vi "RRTAlgorithm2.vi"(0 "Dest x,y":dbl[](array[numeric]), 1 "Robot":T1={"id"=0, "function"=enum."Attacker", "x"=0.0, "y"=0.0, "orientation"=0.0, "v_tangent"=0.0, "v_normal"=0.0, "v_ang"=0.0, "kick_x"=0.0, "kick_z"=0.0, "dribble"=FALSE, "Timestamp"=timestamp(0 s since 1904-01-01), "estimatives"={"est_v_tangent"=0.0, "est_v_normal"=0.0, "est_vx"=0.0, "est_vy"=0.0, "Pos Robot Est"=[], "est_v_ang"=0.0}, "dest_x_kick"=0.0, "dest_y_kick"=0.0, "Gap Coord"=[], "States"=enum."Pass", "Path "=[], "Path  Smooth"=[], "Dest"=[], "vx_desired"=0.0, "vy_desired"=0.0, "slowBehavior"=FALSE, "VSSStates"=enum."Pass", "robotKickState"=enum."none", "role"=enum."DefenderArea"}, 2 "WayPointProb":dbl, 3 "Path in \n(Smooth do Feedback Node)":dbl[][](array[numeric]), 4 "Step":dbl, 5 "GoalProb":dbl, 6 "Simple Path":dbl[][](array[numeric]), 7 "Ball":T10, 8 "Initial Pos x,y":dbl[](array[numeric]), 9 "our_robots":T1[](array[typedef]), 10 "Initial Pos 1,x,y,0":dbl[](array[numeric]), 11 "enemy_robots":T1[](array[typedef]), 12 "ignoreBall?":bool, 13 "Field Geomtery":u32[](array[numeric]), 14 "AttackerAvoidArea":bool=TRUE, 19 "buffer":dbl[](array[numeric])) -> (16 "Path":dbl[][](array[numeric]))   [LabVIEW 2020]
uses:
  Vision_class/Old vision/SSL Detection Frame Simple Estimator Cameras VelCmd Folder/Core/AI Ball.ctl
  Vision_class/Old vision/Controls/AI Robot.ctl
  Vision_class/Old vision/Controls/Functions Enum.ctl
  Controls/estimatives.ctl
  Vision_class/Old vision/Controls/AttackerStates.ctl
  Vision_class/Old vision/Controls/PathDests.ctl
  Vision_class/Old vision/Controls/PathDest.ctl
  Navigation/VSSNavigation/VSSAttackerStates.ctl
  Robot_class/robotKickToStates.ctl
  Robot_class/roles.ctl
  <vilib>/Analysis/_algsub.llb/Real Vector Norm.vi
  <vilib>/Analysis/coordinate.llb/2D Cartesian Coordinate Rotation (Scalar).vi
  <vilib>/Analysis/NI_AALPro.lvlib
panel:
  out "useSimplePath":i32
  out "pathsize":i32
  out "debug":sgl
  out "newTree":dbl[](array[numeric])
  in  "threshold":dbl=80.0
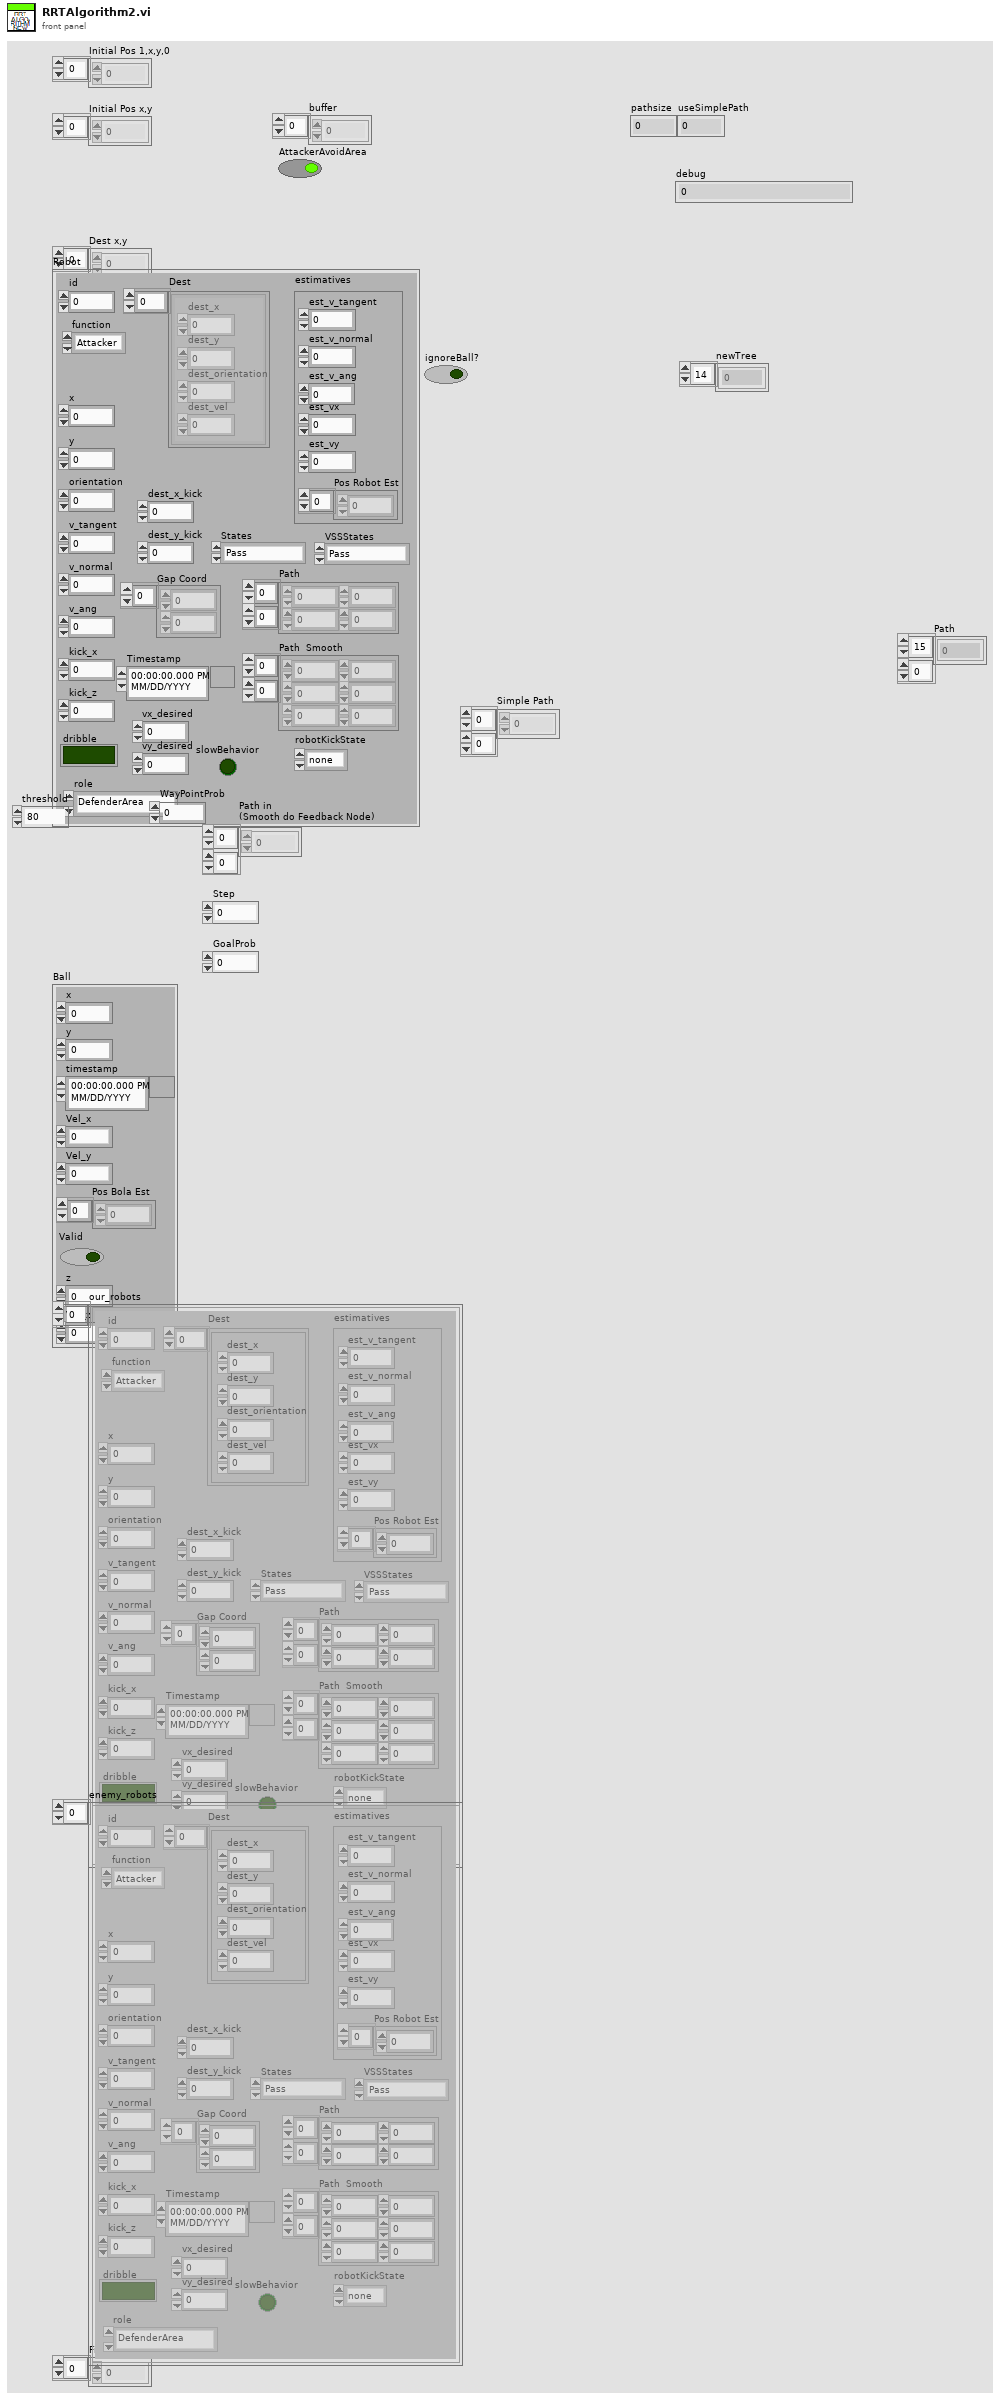
[diagram p1: front panel]
types:
  T1 = typedef "AI Robot.ctl" = cluster{"id":u32, "function":T2, "x":dbl, "y":dbl, "orientation":dbl, "v_tangent":dbl, "v_normal":dbl, "v_ang":dbl, "kick_x":dbl, "kick_z":dbl, "dribble":bool, "Timestamp":timestamp, "estimatives":T3, "dest_x_kick":dbl, "dest_y_kick":dbl, "Gap Coord":dbl[], "States":T4, "Path ":dbl[][], "Path  Smooth":dbl[][], "Dest":T5, "vx_desired":dbl, "vy_desired":dbl, "slowBehavior":bool, "VSSStates":T7, "robotKickState":T8, "role":T9}
  T2 = typedef "Functions Enum.ctl" = enum16{"2nd Striker", "Attacker", "Goalie", "Defender", "Striker", "Goto 0", "Dummy", "Kicker", "ZigZag 0", "ZigZag 1", "ZigZag 2", "ZigZag 3", "ZigZag 4", "ZigZag 5", "ZigZag 6", "ZigZag 7", "ZigZag 8", ""}
  T3 = typedef "estimatives.ctl" = cluster{"est_v_tangent":dbl, "est_v_normal":dbl, "est_vx":dbl, "est_vy":dbl, "Pos Robot Est":dbl[], "est_v_ang":dbl}
  T4 = typedef "AttackerStates.ctl" = enum16{"Pass", "GoToTangent", "BallGetting", "GoToKick", ""}
  T5 = typedef "PathDests.ctl" = T6[]
  T6 = typedef "PathDest.ctl" = cluster{"dest_x":dbl, "dest_y":dbl, "dest_orientation":dbl, "dest_vel":dbl}
  T7 = typedef "VSSAttackerStates.ctl" = enum16{"Pass", "GoToTangent", "BallGetting", "GoToKick", "Rotate anti-clockwise", "Rotate Clockwise", ""}
  T8 = typedef "robotKickToStates.ctl" = enum16{"shootFromDirect", "avoidCollideBall", "goToBackBall", "none", "walk", "turn", "oldKickToShoot", "oldKickToGoToBackBall", "shoot"}
  T9 = typedef "roles.ctl" = enum16{"SimpleBallPlacement", "BallPlacementAllyPasser", "BallPlacementAllyReceiver", "BallPlacementEnemy", "5Robots5th", "PassBestReceiver", "5Robots4th", "5Robots3rd", "5Robots2nd", "5Robots1st", "PassBestRobot", "WaitPass", "ABCThirdKicker", "ABCFirstKicker", "ABCSecondKicker", "Tabler", "TableFinalizer", "PrepareRollToPassRoller", "PrepareRollToPassReceiver", "SimplePassRoll", "SimplePassRollReceiver", "PenaltyDefense", "PreparePassReceiver 2", "PreparePassReceiver 1", "PassObserver", "Timeout", "Goto", "ZigZag", "None", "BallOutOfField", "DefenderArea", "Duelist", "AttackerStop", "FollowAttacker", "KeeperRole", "KickPenalty", "AttackerAimGoal", "AttackerBlock", "Marker", "Halt", "Shoot", "PassKicker", "PassReceiver", "TestRole", "PenaltyAttacker"}
  T10 = typedef "AI Ball.ctl" = cluster{"x":dbl, "y":dbl, "timestamp":timestamp, "Vel_x":dbl, "Vel_y":dbl, "Pos Bola Est":dbl[], "Valid":bool, "z":dbl, "Vel_z":dbl}
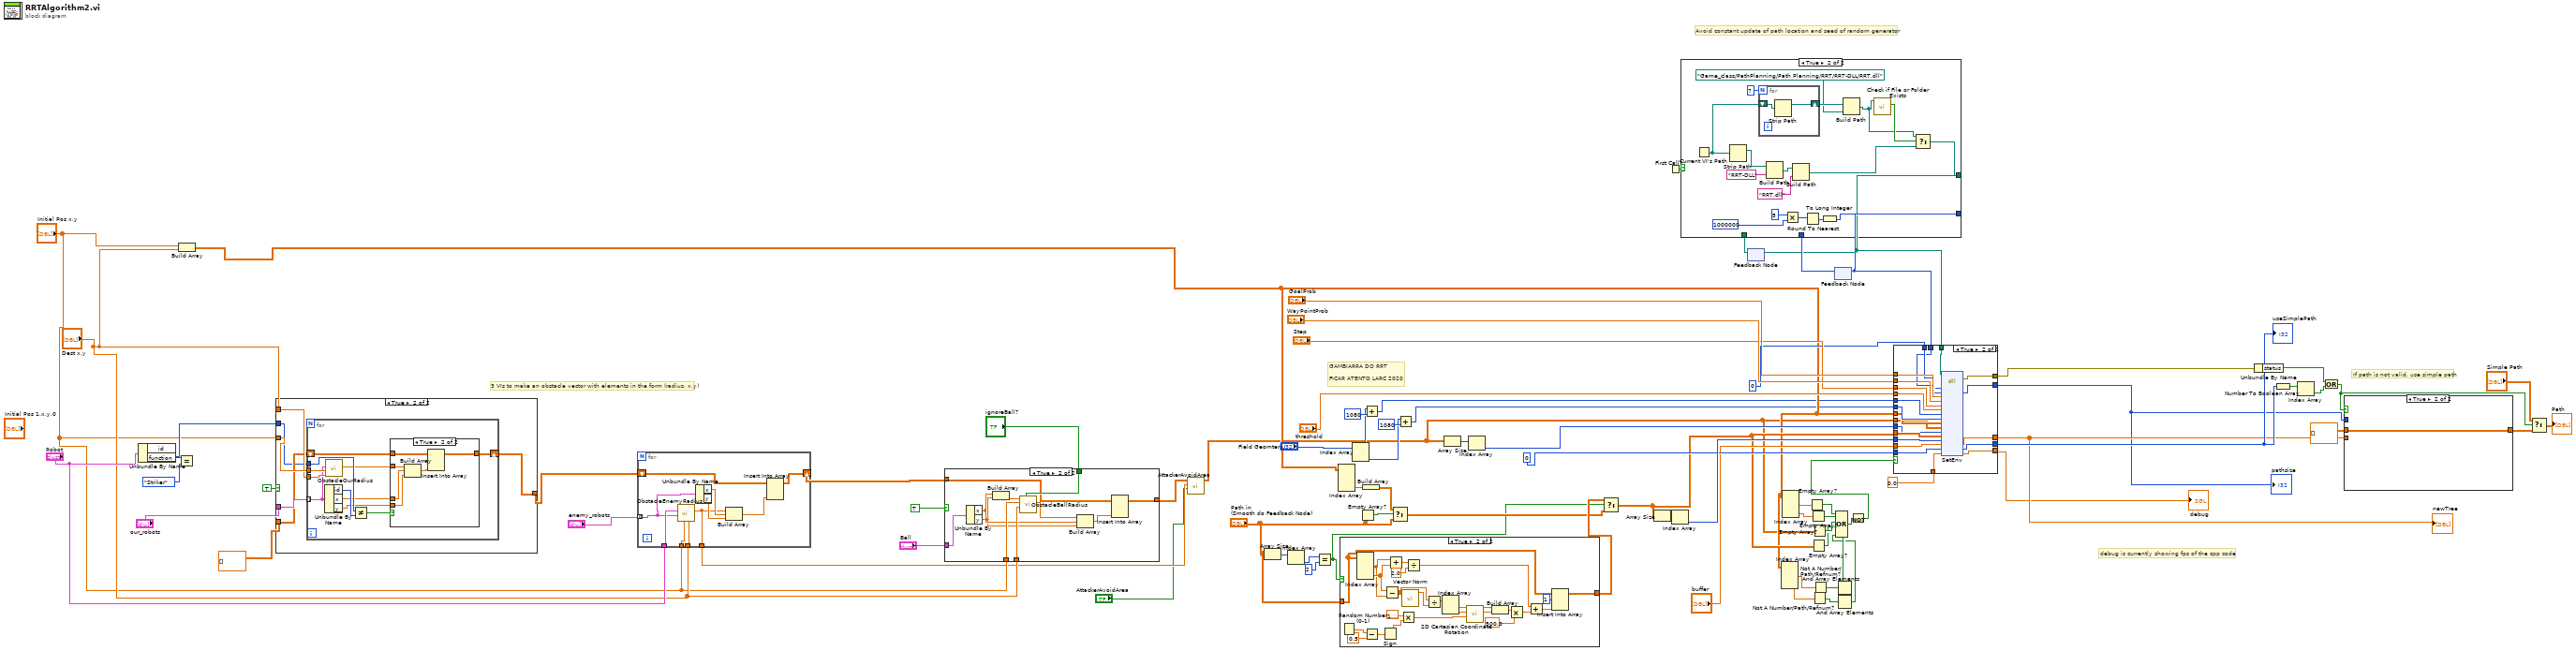
[diagram p0: block diagram]
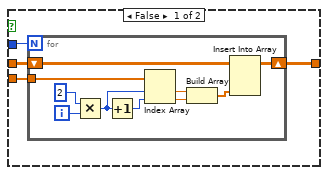
[diagram p4: hidden frame]
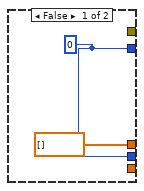
[diagram p5: hidden frame]
diagram:
  # "GAMBIARRA DO RRT\n\nFICAR ATENTO LARC 2020"
  # "debug is currently showing fps of the cpp code"
  # "If path is not valid, use simple path"
  # "3 VIs to make an obstacle vector with elements in the form (radius, x,y)"
  # "Avoid constant update of path location and seed of random generator"
  n1 = Unbundle By Name("Robot") -> ("id"=w69:u32, "function"=w73:T2)
  n2 = Equal?(x=w73, y=Functions_Enum."Striker" ("function")) -> ()  [unwired: 1 out]
  n3 = Build Array("Initial Pos x,y", "Dest x,y") -> (w12:dbl[][])
  n4 = case shown="True" TRUE {
    tunnel: "our_robots" -> [_ w89]
    tunnel: "Initial Pos x,y" -> [_ w88]
    tunnel: "Dest x,y" -> [_ w87]
    tunnel: dbl[][] [] ("appended array") -> [w83 w86]
    tunnel: [w83 w84] -> w66
    tunnel: w69 -> [_ w85]
    frame False {
    }
    frame True {
      n5 = for {
        tunnel: w89 -> [w98] mode=indexing
        tunnel: w88 -> [w100]
        tunnel: w87 -> [w99]
        shift-right: [w90] -> w84
        shift-left: w86 -> [w94]
        tunnel: w85 -> [w96]
        n6 = Unbundle By Name(w98) -> ("id"=w97:u32, "x"=w92:dbl, "y"=w91:dbl)
        n7 = call "ObstacleOurRadius.vi"("Goal"=w99, "Initial State"=w100, "other robot"=w98) -> ("obstacle enemy radius"=w93:dbl)  [unwired: 8 in]
        n8 = Not Equal?(x=w96, y=w97) -> (x != y?=w95:bool)
        n9 = case shown="True" w95 {
          tunnel: w94 -> [w101 w104]
          tunnel: [w101 w102] -> w90
          tunnel: w93 -> [_ w107]
          tunnel: w92 -> [_ w106]
          tunnel: w91 -> [_ w105]
          frame False {
          }
          frame True {
            n10 = Build Array(w107, w106, w105) -> (w103:dbl[])
            n11 = Insert Into Array(array=w104, new element=w103) -> (w102:dbl[][])  [unwired: 2 in]
          }
        }
      }
    }
  }
  n12 = for {
    tunnel: "enemy_robots" -> [w114] mode=indexing
    tunnel: "Initial Pos x,y" -> [w117]
    tunnel: "Dest x,y" -> [w116]
    tunnel: "Robot" -> [w115]
    shift-right: [w109] -> w62
    shift-left: w66 -> [w111]
    tunnel: [w108] -> w2
    n13 = call "ObstacleEnemyRadius.vi"("Goal"=w116, "Initial State"=w117, "Robot enemy"=w114, "Robot in"=w115) -> ("obstacle enemy radius"=w108:dbl)  [unwired: 7 in]
    n14 = Unbundle By Name(w114) -> ("x"=w113:dbl, "y"=w112:dbl)
    n15 = Build Array(w108, w113, w112) -> (w110:dbl[])
    n16 = Insert Into Array(array=w111, new element=w110) -> (w109:dbl[][])  [unwired: 2 in]
  }
  n17 = case shown="True" TRUE {
    tunnel: "Ball" -> [_ w129]
    tunnel: "Initial Pos x,y" -> [_ w127]
    tunnel: "Dest x,y" -> [_ w126]
    tunnel: "ignoreBall?" -> [_ w125]
    tunnel: w62 -> [w118 w124]
    tunnel: [w118 w123] -> w3
    frame False {
    }
    frame True {
      n18 = Unbundle By Name(w129) -> ("x"=w121:dbl, "y"=w120:dbl)
      n19 = Build Array(w121, w120) -> (w128:dbl[])
      n20 = call "ObstacleBallRadius.vi"("ignoreBall?"=w125, "Goal"=w126, "Initial State"=w127, "ball"=w128) -> ("obstacle enemy radius"=w122:dbl)  [unwired: 7 in]
      n21 = Build Array(w122, w121, w120) -> (w119:dbl[])
      n22 = Insert Into Array(array=w124, new element=w119) -> (w123:dbl[][])  [unwired: 2 in]
    }
  }
  n23 = call "AttackerAvoidArea.vi"("AttackerAvoidArea"="AttackerAvoidArea", "obstacle enemy radius"=w2, "array in"=w3) -> ("array out"=w4:dbl[][])  [unwired: 8 in]
  n24 = Array Size(array="Path in \n(Smooth do Feedback Node)") -> (size(s)=w40:i32[])
  n25 = Index Array(array=w40) -> (element=w39:i32)  [unwired: 1 in]
  n26 = Equal?(x=w39, y=2) -> (x = y?=w34:bool)
  n27 = Index Array(array=w12) -> (element #2=w57:dbl[])  [unwired: 4 in, 1 out]
  n28 = case shown="True" w34 {
    tunnel: "Path in \n(Smooth do Feedback Node)" -> [w130 w137]
    tunnel: [w130 w134] -> w36
    frame False {
    }
    frame True {
      n29 = Random Number (0-1)() -> (number: 0 to 1=w131:dbl)
      n30 = Index Array(array=w137) -> (element #1=w152:dbl[], element #2=w153:dbl[])  [unwired: 4 in]
      n31 = Subtract(x=w131, y=0.5) -> (x-y=w133:dbl)
      n32 = Sign(1:w133) -> (0:w148:dbl)
      n33 = Subtract(x=w153, y=w152) -> (x-y=w150:dbl[])
      n34 = Add(x=w152, y=w153) -> (x+y=w155:dbl[])
      n35 = Multiply(x=1.5707963267948966, y=w148) -> (x*y=w147:dbl)
      n36 = call-poly <vilib>:"Vector Norm.vi"("Input Vector"=w150) -> ("norm"=w151:dbl)  [unwired: 9 in, 1 out]
      n37 = Divide(x=w155, y=2.0) -> (x/y=w138:dbl[])
      n38 = Divide(x=w150, y=w151) -> (x/y=w146:dbl[])
      n39 = Index Array(array=w146) -> (element #1=w145:dbl, element #2=w144:dbl)  [unwired: 2 in]
      n40 = call-poly <vilib>:"2D Cartesian Coordinate Rotation.vi"("theta"=w147, "y"=w144, "x"=w145) -> ("y out"=w142:dbl, "x out"=w143:dbl)  [unwired: 6 in, 1 out]
      n41 = Build Array(w143, w142) -> (w140:dbl[])
      n42 = Multiply(x=w140, y=500.0) -> (x*y=w139:dbl[])
      n43 = Add(x=w138, y=w139) -> (x+y=w135:dbl[])
      n44 = Insert Into Array(array=w137, index (row)=1, new element=w135) -> (w134:dbl[][])  [unwired: 1 in]
    }
  }
  n45 = Index Array(array="Field Geomtery") -> (element #1=w7:u32, element #2=w10:u32)  [unwired: 2 in]
  n46 = Empty Array?(array="Path in \n(Smooth do Feedback Node)") -> (empty?=w58:bool)
  n47 = Build Array(w57) -> (w50:dbl[][])
  n48 = Add(x=w7, y=u32 1080) -> (x+y=w6:u32)
  n49 = Select(t=w50, s=w58, f="Path in \n(Smooth do Feedback Node)") -> (s? t:f=w35:dbl[][])
  n50 = Add(x=w10, y=u32 1080) -> (x+y=w9:u32)
  n51 = Array Size(array=w4) -> (size(s)=w60:i32[])
  n52 = Index Array(array=w60) -> (element=w76:i32)  [unwired: 1 in]
  n53 = Select(t=w36, s=w34, f=w35) -> (s? t:f=w30:dbl[][])
  n54 = Array Size(array=w30) -> (size(s)=w59:i32[])
  n55 = First Call?() -> (First Call?: T/F=w47:bool)
  n56 = Index Array(array=w59) -> (element=w78:i32)  [unwired: 1 in]
  n57 = feedback #1() -> (w46:path)  [unwired: 1 in]
  n58 = Index Array(array=w12) -> (element #1=w19:dbl[], element #2=w18:dbl[])  [unwired: 4 in]
  n59 = Index Array(array=w12) -> (element #1=w32:dbl[], element #2=w31:dbl[])  [unwired: 4 in]
  n60 = Empty Array?(array=w32) -> (empty?=w21:bool)
  n61 = Empty Array?(array=w31) -> (empty?=w20:bool)
  n62 = Empty Array?(array=w30) -> (empty?=w28:bool)
  n63 = Empty Array?(array=w4) -> (empty?=w29:bool)
  n64 = Not A Number/Path/Refnum?(number/path/refnum=w18) -> (NaN/Path/Refnum?=w16:bool[])
  n65 = Not A Number/Path/Refnum?(number/path/refnum=w19) -> (NaN/Path/Refnum?=w17:bool[])
  n66 = feedback #2() -> (w44:i32)  [unwired: 1 in]
  n67 = case shown="True" w47 {
    tunnel: [w157 w161] -> w42
    tunnel: w46 -> [w157 _]
    tunnel: [w156 w169] -> w43
    tunnel: w44 -> [w156 _]
    frame False {
    }
    frame True {
      n68 = Current VI's Path() -> (path=w165:path)
      n69 = Strip Path(path=w165) -> (stripped path=w174:path)  [unwired: 1 out]
      n70 = for {
        N: 7 -> [_]
        shift-right: [w175] -> w163
        shift-left: w165 -> [w176]
        n71 = Strip Path(path=w176) -> (stripped path=w175:path)  [unwired: 1 out]
      }
      n72 = Build Path(base path=w174, name or relative path="RRT-DLL") -> (appended path=w167:path)
      n73 = Multiply(x=5, y=1000000) -> (x*y=w171:i32)
      n74 = Build Path(base path=w167, name or relative path="RRT.dll") -> (appended path=w158:path)
      n75 = Round To Nearest(number=w171) -> (nearest integer value=w170:i32)
      n76 = To Long Integer(number=w170) -> (32bit integer=w169:i32)
      n77 = Build Path(base path=w163, name or relative path=path "Game_class/PathPlanning/Path Planning/RRT/RRT-DLL/RRT.dll") -> (appended path=w159:path)
      n78 = call <vilib>:"Check if File or Folder Exists.vi"("path"=w159) -> ("file or folder exists?"=w160:bool)  [unwired: 8 in, 2 out]
      n79 = Select(t=w159, s=w160, f=w158) -> (s? t:f=w161:path)
    }
  }
  n80 = feedback-in #1(w42) -> ()
  n81 = feedback-in #2(w43) -> ()
  n82 = And Array Elements(Boolean array=w17) -> (logical AND=w15:bool)
  n83 = And Array Elements(Boolean array=w16) -> (logical AND=w14:bool)
  n84 = Compound Arithmetic op=OR(w21, w20, w29, w28, w15, w14) -> (w27:bool)
  n85 = Not(x=w27) -> (.not. x?=w13:bool)
  n86 = case shown="True" w13 {
    tunnel: "GoalProb" -> [_ w200]
    tunnel: "WayPointProb" -> [_ w199]
    tunnel: "Step" -> [_ w198]
    tunnel: "threshold" -> [_ w197]
    tunnel: w6 -> [_ w196]
    tunnel: w9 -> [_ w195]
    tunnel: w12 -> [_ w194]
    tunnel: w4 -> [_ w193]
    tunnel: w30 -> [_ w192]
    tunnel: w78 -> [_ w191]
    tunnel: 0 -> [_ w190]
    tunnel: "buffer" -> [_ w189]
    tunnel: [dbl[] [] ("newTree") w188] -> w74
    tunnel: [w177 w187] -> w75
    tunnel: [w177 w180] -> w41
    tunnel: w76 -> [_ w186]
    tunnel: sgl 0.0 ("debug") -> [_ w184]
    tunnel: 0 -> [_ w185]
    tunnel: [_ w183] -> w45
    tunnel: w43 -> [_ w182]
    tunnel: w42 -> [_ w181]
    tunnel: [_ w179] -> w26
    frame False {
      w177 = 0 ("pathsize")
    }
    frame True {
      n87 = dll-call lib="C:/Users/anton/source/repos/RRT/x64/Release/RRT.dll" fn="SetEnv"(path in=w181, "seed"=w182, "pathsize"=w185, "probGoal"=w200, "probWaypoint"=w199, "step"=w198, "threshold"=w197, "field_length"=w196, "field_width"=w195, "Start/End"=w194, "obsList"=w193, "obsLen"=w186, "lastTree"=w192, "lastTreeLen"=w191, "newTree"=w189, "useSimplePath"=w190, "debug"=w184) -> (error out=w179:errorcluster, "pathsize"=w180:i32, "newTree"=w188:sgl[], "useSimplePath"=w187:i8, "debug"=w183:sgl)  [unwired: 15 in, 1 out]
    }
  }
  "newTree" <- w74
  "debug" <- w45
  "pathsize" <- w41
  "useSimplePath" <- w75
  n88 = Unbundle By Name(w26) -> ("status"=w24:bool)
  n89 = Number To Boolean Array(number=w75) -> (Boolean array=w53:bool[])
  n90 = Index Array(array=w53) -> (element=w25:bool)  [unwired: 1 in]
  n91 = Or(x=w24, y=w25) -> (x .or. y?=w23:bool)
  n92 = case shown="True" w23 {
    tunnel: w74 -> [w204 _]
    tunnel: dbl[][] [] ("s? t:f") -> [w203 w215]
    tunnel: w41 -> [w202 _]
    tunnel: [w201 w215] -> w54
    frame False {
      n93 = for {
        N: w202 -> [_]
        tunnel: w204 -> [w212]
        shift-right: [w205] -> w201
        shift-left: w203 -> [w207]
        i -> [w214]
        n94 = Multiply(x=2, y=w214) -> (x*y=w210:i32)
        n95 = Increment(x=w210) -> (x+1=w211:i32)
        n96 = Index Array(array=w212, index #1=w210, index #2=w211) -> (element #1=w209:dbl, element #2=w208:dbl)
        n97 = Build Array(w209, w208) -> (w206:dbl[])
        n98 = Insert Into Array(array=w207, new element=w206) -> (w205:dbl[][])  [unwired: 2 in]
      }
    }
    frame True {
    }
  }
  n99 = Select(t="Simple Path", s=w23, f=w54) -> (s? t:f=→"Path":dbl[][])
